vi "internetCheck.vi"(2 "error in (no error)":errorcluster) -> (0 "error out":errorcluster, 1 "Status":bool)   [LabVIEW 2021]
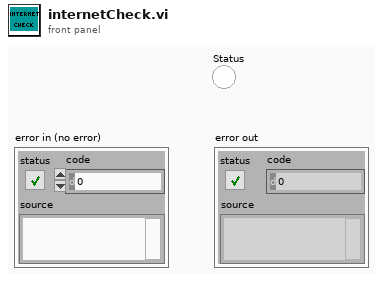
[diagram p1: front panel]
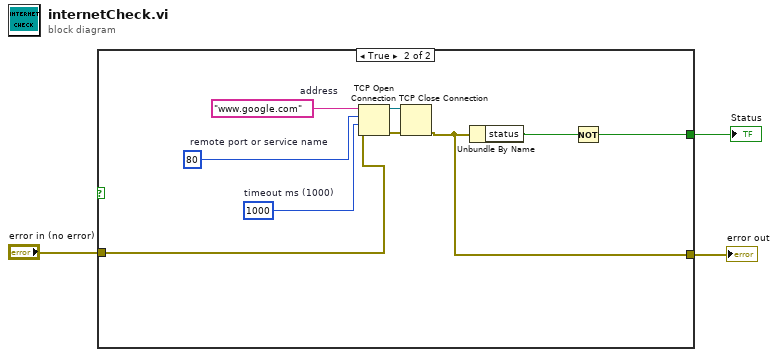
[diagram p0: block diagram]
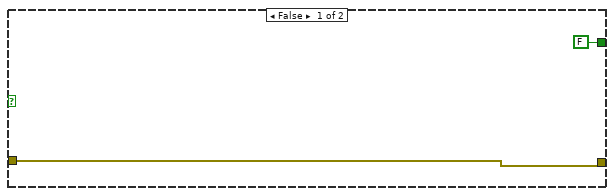
[diagram p2: hidden frame]
diagram:
  n1 = case shown="\"No error\"" {
    selector: _ -> [_ _]
    tunnel: "error in (no error)" -> [w5 w8]
    tunnel: [w5 w7] -> w2
    tunnel: [FALSE w6] -> w3
    frame False {
    }
    frame True {
      w10 = 1000  # timeout ms (1000)
      w11 = u16 80  # remote port or service name
      w12 = "www.google.com"  # address
      n2 = TCP Open Connection(address=w12, remote port or service name=w11, timeout ms (60000)=w10, error in (no error)=w8) -> (connection ID=w14:refnum<k5>, error out=w13:errorcluster)  [unwired: 1 in]
      n3 = TCP Close Connection(connection ID=w14, error in (no error)=w13) -> (error out=w7:errorcluster)  [unwired: 1 in, 1 out]
      n4 = Unbundle By Name(w7) -> ("status"=w9:bool)
      n5 = Not(x=w9) -> (.not. x?=w6:bool)
    }
  }
  "error out" <- w2
  "Status" <- w3
